vi "006 System Gloabl.vi"() -> ()   [LabVIEW 2020]
panel:
  in  "RootPath":path
  in  "Load_Model":string="NBT_V1.0.0"
  in  "Mode":enum16{"Release", "Debug"}(ring)
  in  "Version":string="V1.0"
  in  "Project":string="0001_HZKD_ST01"
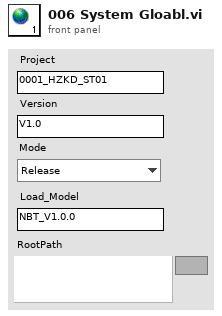
[diagram p1: front panel]
diagram:
